vi "to and from repo test.vi"() -> ()   [LabVIEW 2013, in "configuration tests.lvlib"]
uses:
  configuration tests.lvlib
  Framework Configuration Classes/platypus configuration/targets cluster.ctl
  Framework Configuration Classes/target configuration/PL_Target Configuration.lvclass
  Framework Configuration Classes/platypus configuration/engines cluster.ctl
  <vilib>/NI/Module Execution Interface/Engine Configuration/engine configuration.lvclass
  <vilib>/NI/Tag Bus Module Framework/module configuration/TBM module configuration.lvclass
  Framework Configuration Classes/platypus configuration/systems cluster.ctl
  Framework Configuration Classes/system configuration/PL_System Configuration.lvclass
  Configuration Editor/Classes/SystemConfigRepo/SystemConfigRepo.lvclass
  Framework Configuration Classes/class cache/cache definition.ctl
  Framework Configuration Classes/class cache/cache search configuration.ctl
  Framework Configuration Classes/class cache/cached class information.ctl
  Framework Configuration Classes/class cache/target class metadata.ctl
  Framework Configuration Classes/class cache/class metadata.ctl
  <vilib>/NI/Tag Bus Module Framework/root configuration/Target Types.ctl
  <vilib>/NI/Tag Bus/tag/Data Type.ctl
  <vilib>/NI/Tag Bus/tag/tag descriptor.lvclass
  <vilib>/NI/Configuration Framework/serializable configuration/NISE_CEF_serializable configuration.lvclass/NISE_CEF_serializable configuration.ctl
  <vilib>/NI/Configuration Framework/serializable configuration/NISE_CEF_serializable configuration.lvclass
  Framework Configuration Classes/target configuration/PL_Target Configuration.lvclass/PL_Target Configuration.ctl
  Framework Configuration Classes/system configuration/PL_System Configuration.lvclass/PL_System Configuration.ctl
  test module/module/configuration/TEST CONFIGURATION.lvclass
  test module/module/configuration/state module configuration.ctl
  <vilib>/NI/Tag Bus Module Framework/channel/TBM channel.lvclass
  test module/module/configuration/TEST CONFIGURATION.lvclass/TEST CONFIGURATION.ctl
  Configuration Editor/Classes/SystemConfigRepo/SystemConfigRepo.lvclass/SystemConfigRepo.ctl
  <vilib>/NI/Tag Bus/tag/tag descriptor.lvclass/tag descriptor.ctl
  test module/module/configuration/Write state module configuration.vi
  test module/module/configuration/Read state module configuration.vi
  <vilib>/NI/Tag Bus/tag/read tag name.vi
  Framework Configuration Classes/target configuration/Write name.vi
  Framework Configuration Classes/system configuration/Write Configuration Name.vi
  Framework Configuration Classes/system configuration/Write save time.vi
  Configuration Editor/Classes/SystemConfigRepo/Write Systems.vi
  Configuration Editor/Classes/SystemConfigRepo/Read Systems.vi
  Framework Configuration Classes/system configuration/Read Configuration Name.vi
  Framework Configuration Classes/system configuration/Read save time.vi
  Framework Configuration Classes/target configuration/Read name.vi
  Framework Configuration Classes/platypus configuration/PLConfigurationSerializer.lvlib
  Framework Configuration Classes/class cache/PL_class cache.lvlib
  <vilib>/NI/Tag Bus Module Framework/root configuration/TBM configuration.lvclass
panel:
  out "moduleok":bool
  out "engok":bool
  out "engclasserr":errorcluster
  out "targok":bool
  out "sysok":bool
  # "THIS TEST FAILS WITHOUT A SAMPLE ENGINE IMPLEMENTATION"
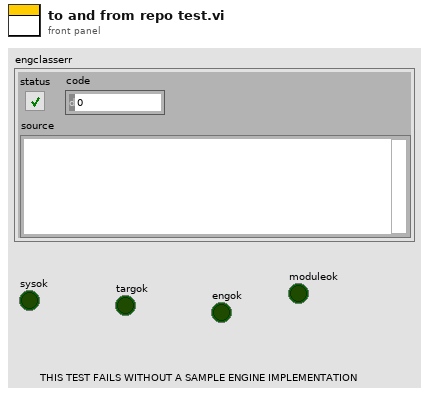
[diagram p1: front panel]
types:
  T1 = typedef "PLConfigurationSerializer.lvlib/engines cluster.ctl" = cluster{"engine configuration":refnum<class "engine configuration.lvclass">, "modules":refnum<class "TBM module configuration.lvclass">[]}
  T2 = typedef "PLConfigurationSerializer.lvlib/systems cluster.ctl" = cluster{"System Configuration":refnum<class "PL_System Configuration.lvclass">, "targets":T3[]}
  T3 = typedef "PLConfigurationSerializer.lvlib/targets cluster.ctl" = cluster{"Target Configuration":refnum<class "PL_Target Configuration.lvclass">, "engines":T1[]}
  T4 = typedef "PL_class cache.lvlib/cache definition.ctl" = cluster{"configuration":T5, "class cache data":T6}
  T5 = typedef "PL_class cache.lvlib/cache search configuration.ctl" = cluster{"Search Paths":path[], "Folders to Exclude":string[], "full class list":path[]}
  T6 = typedef "PL_class cache.lvlib/cached class information.ctl" = cluster{"targets":T7[], "engines":T8[], "modules":T8[], "ignored class list":path[]}
  T7 = typedef "PL_class cache.lvlib/target class metadata.ctl" = cluster{"file name":string, "fully qualified name":string, "menu display name":string, "configuration class name":string}
  T8 = typedef "PL_class cache.lvlib/class metadata.ctl" = cluster{"file name":string, "fully qualified name":string, "menu display name":string, "configuration class":string, "instances allowed":i32, "supported targets":T9[]}
  T9 = typedef "TBM configuration.lvclass/Target Types.ctl" = enum16{"Windows", "Mac", "Linux", "Linux RT ARM", "VxWorks", "Pharlap", "Other", "Linux RT x64"}
  T10 = typedef "tag bus.lvlib/tag descriptor.lvclass/Data Type.ctl" = enum16{"Double", "Single", "I64", "I32", "I16", "I8", "U64", "U32", "U16", "U8", "Boolean", "String", "Array of Double", "Array of Single", "Array of I64", "Array of I32", "Array of I16", "Array of I8", "Array of U64", "Array of U32", "Array of U16", "Array of U8", "Array of Boolean", "Array of String"}
  T11 = typedef "configuration tests.lvlib/TEST CONFIGURATION.lvclass/state module configuration.ctl" = cluster{"fixed input":refnum<class "TBM channel.lvclass">, "fixed output":refnum<class "TBM channel.lvclass">, "initial state":u8}
  T12 = typedef "NISE_CEF_Node.lvclass/NodeRef.ctl" = refnum<data-value>
  T13 = typedef "user tag bus module configuration.lvclass/state module configuration.ctl" = cluster{"fixed input":refnum<class "TBM channel.lvclass">, "fixed output":refnum<class "TBM channel.lvclass">, "initial state":u8}
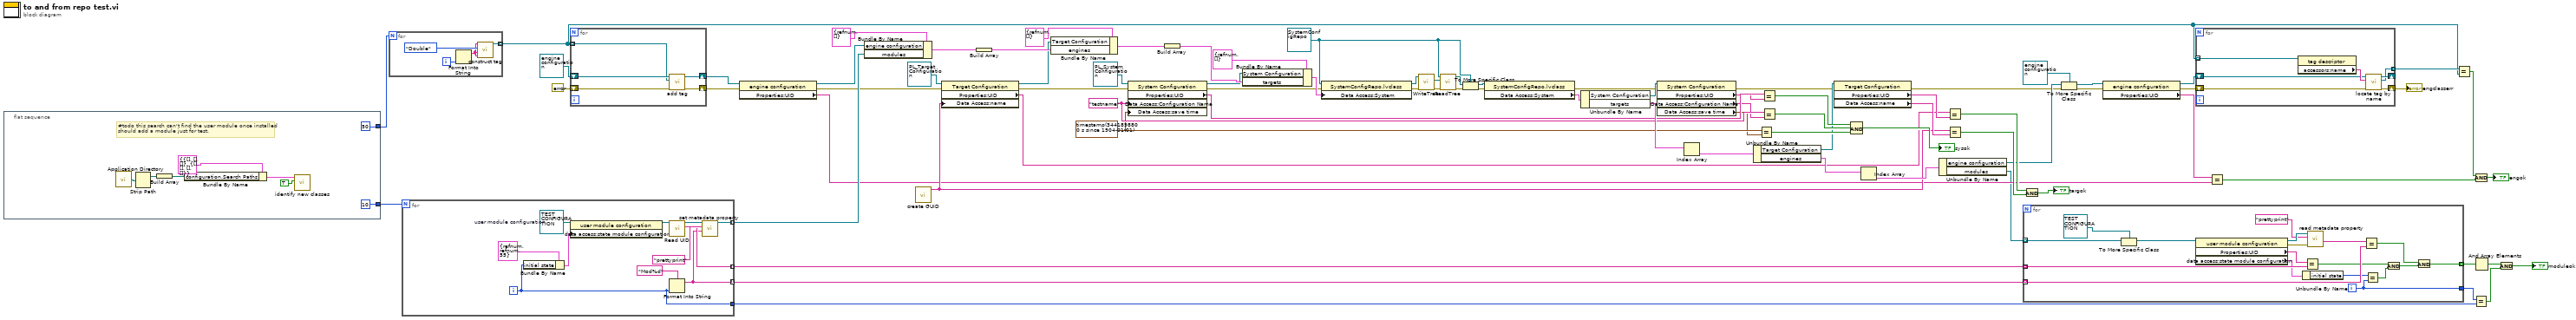
[diagram p0: block diagram]
diagram:
  w26 = refnum<class "SystemConfigRepo.lvclass"> refnum ("SystemConfigRepo in")
  w62 = timestamp(3441898800 s since 1904-01-01) ("save time")
  w63 = "testname" ("Configuration Name")
  n1 = flat-sequence {
    tunnel: [10] -> w22
    tunnel: [50] -> w1
    frame #0 {
      # "#todo this search can't find the user module once installed\nshould add a module just for test."
      n2 = call <vilib>:"Application Directory.vi"() -> ("Application Directory"=w83:path)
      n3 = Strip Path(path=w83) -> (stripped path=w84:path)  [unwired: 1 out]
      n4 = Build Array(w84) -> (w85:path[])
      n5 = Bundle By Name(cluster=T4 {"configuration"={"Search Paths"=[], "Folders to Exclude"=[], "full class list"=[]}, "class cache data"={"targets"=[], "engines"=[], "modules"=[], "ignored class list"=[]}} ("cache"), "configuration.Search Paths"=w85) -> (w89:T4)
      n6 = call "identify new classes.vi"("force scan"=TRUE, "cache in"=w89) -> ()  [unwired: 8 in, 2 out]
    }
  }
  n7 = for {
    N: w1 -> [_]
    tunnel: [w91] -> w6 mode=indexing
    i -> [w94]
    n8 = Format Into String(w94) -> (resulting string=w92:string)  [unwired: 3 in, 1 out]
    n9 = call <vilib>:"construct tag.vi"("raw default"=w92, "metadata"=w92, "data type"=Data_Type."Double", "name"=w92) -> ("system tag out"=w91:refnum<class "tag descriptor.lvclass">)  [unwired: 6 in, 1 out]
  }
  n10 = for {
    N: w22 -> [_]
    tunnel: [w103] -> w75 mode=indexing
    tunnel: [w101] -> w36 mode=indexing
    tunnel: [w100] -> w37 mode=indexing
    tunnel: [w95] -> w2
    i -> [w95]
    w99 = refnum<class "TEST CONFIGURATION.lvclass"> refnum  # user module configuration
    n11 = Bundle By Name(cluster=T11 {"fixed input"=refnum, "fixed output"=refnum, "initial state"=55} ("state module configuration"), "initial state"=w95) -> (w96:T11)
    n12 = property class="user module configuration"(reference=w99, "data access:state module configuration"=w96) -> (reference out=w98:refnum<class "TEST CONFIGURATION.lvclass">)  [unwired: 1 in, 1 out]
    n13 = call <vilib>:"Read UID.vi"("configuration in"=w98) -> ("instance id"=w101:string, "configuration out"=w104:refnum<class "TEST CONFIGURATION.lvclass">)  [unwired: 8 in, 1 out]
    n14 = Format Into String(format string="Mod%d", w95) -> (resulting string=w100:string)  [unwired: 2 in, 1 out]
    n15 = call <vilib>:"set metadata property.vi"("value"=w100, "key"="prettyprint", "configuration in"=w104) -> ("configuration out"=w103:refnum<class "TEST CONFIGURATION.lvclass">)  [unwired: 7 in, 1 out]
  }
  n16 = for {
    shift-right: [w110] -> w10
    shift-left: refnum<class "engine configuration.lvclass"> refnum ("Engine Configuration") -> [w109]
    shift-right: [w108] -> w8
    shift-left: errorcluster {"status"=FALSE, "code"=0, "source"=""} ("error out") -> [w107]
    tunnel: w6 -> [w106] mode=indexing
    n17 = call <vilib>:"add tag.vi"("error in"=w107, "tag descriptor"=w106, "engine configuration in"=w109) -> ("error out"=w108:errorcluster, "engine configuration out"=w110:refnum<class "engine configuration.lvclass">)  [unwired: 7 in]
  }
  n18 = property class="engine configuration"(reference=w10, error in=w8) -> (reference out=w74:refnum<class "engine configuration.lvclass">, error out=w17:errorcluster, "Properties:UID"=w39:string)
  n19 = Bundle By Name(cluster=T1 {"engine configuration"=refnum, "modules"=[]} ("engines cluster"), "engine configuration"=w74, "modules"=w75) -> (w81:T1)
  n20 = call <vilib>:"create GUID.vi"() -> ("uuid"=w48:string)  [unwired: 11 in]
  n21 = property class="Target Configuration"(reference=refnum<class "PL_Target Configuration.lvclass"> refnum ("Target Configuration"), error in=w17, "Data Access:name"=w48) -> (reference out=w72:refnum<class "PL_Target Configuration.lvclass">, error out=w16:errorcluster, "Properties:UID"=w47:string)
  n22 = Build Array(w81) -> (w79:T1[])
  n23 = Bundle By Name(cluster=T3 {"Target Configuration"=refnum, "engines"=[]} ("targets cluster"), "Target Configuration"=w72, "engines"=w79) -> (w78:T3)
  n24 = property class="System Configuration"(reference=refnum<class "PL_System Configuration.lvclass"> refnum ("System Configuration"), error in=w16, "Data Access:Configuration Name"=w63, "Data Access:save time"=w62) -> (reference out=w70:refnum<class "PL_System Configuration.lvclass">, error out=w18:errorcluster, "Properties:UID"=w64:string)
  n25 = Build Array(w78) -> (w76:T3[])
  n26 = Bundle By Name(cluster=T2 {"System Configuration"=refnum, "targets"=[]} ("system"), "System Configuration"=w70, "targets"=w76) -> (w31:T2)
  n27 = property class="SystemConfigRepo.lvclass"(reference=w26, error in=w18, "Data Access:System"=w31) -> (reference out=w33:refnum<class "SystemConfigRepo.lvclass">, error out=w32:errorcluster)
  n28 = call-dynamic "WriteTree.vi"("error in"=w32, "SystemConfigRepo in"=w33) -> ("error out"=w30:errorcluster, "root"=w29:T12)  [unwired: 7 in, 1 out]
  n29 = call-dynamic "ReadTree.vi"("error in"=w30, "root"=w29, "SystemConfigRepo in"=w26) -> ("error out"=w23:errorcluster, "repository out"=w28:refnum<class "NISE_CEF_Repository.lvclass">)  [unwired: 7 in]
  n30 = To More Specific Class(target class=w26, reference=w28, error in=w23) -> (specific class reference=w27:refnum<class "SystemConfigRepo.lvclass">, error out=w24:errorcluster)
  n31 = property class="SystemConfigRepo.lvclass"(reference=w27, error in=w24) -> (error out=w19:errorcluster, "Data Access:System"=w25:T2)  [unwired: 1 out]
  n32 = Unbundle By Name(w25) -> ("System Configuration"=w65:refnum<class "PL_System Configuration.lvclass">, "targets"=w69:T3[])
  n33 = property class="System Configuration"(reference=w65, error in=w19) -> (error out=w20:errorcluster, "Properties:UID"=w59:string, "Data Access:Configuration Name"=w60:string, "Data Access:save time"=w61:timestamp)  [unwired: 1 out]
  n34 = Index Array(array=w69) -> (element=w67:T3)  [unwired: 1 in]
  n35 = Unbundle By Name(w67) -> ("Target Configuration"=w54:refnum<class "PL_Target Configuration.lvclass">, "engines"=w68:T1[])
  n36 = Equal?(x=w62, y=w61) -> (x = y?=w56:bool)
  n37 = Equal?(x=w64, y=w59) -> (x = y?=w58:bool)
  n38 = Equal?(x=w63, y=w60) -> (x = y?=w57:bool)
  n39 = property class="Target Configuration"(reference=w54, error in=w20) -> (error out=w21:errorcluster, "Properties:UID"=w49:string, "Data Access:name"=w50:string)  [unwired: 1 out]
  n40 = Compound Arithmetic op=AND(w58, w57, w56) -> (→"sysok":bool)
  n41 = Index Array(array=w68) -> (element=w66:T1)  [unwired: 1 in]
  n42 = Unbundle By Name(w66) -> ("engine configuration"=w46:refnum<class "engine configuration.lvclass">, "modules"=w38:refnum<class "TBM module configuration.lvclass">[])
  n43 = Equal?(x=w47, y=w49) -> (x = y?=w51:bool)
  n44 = Equal?(x=w48, y=w50) -> (x = y?=w52:bool)
  n45 = for {
    tunnel: w38 -> [w128] mode=indexing
    tunnel: w37 -> [w123] mode=indexing
    tunnel: w36 -> [w121] mode=indexing
    tunnel: [w119] -> w35 mode=indexing
    tunnel: [w111] -> w4
    i -> [w111]
    n46 = To More Specific Class(target class=refnum<class "TEST CONFIGURATION.lvclass"> refnum ("user module configuration"), reference=w128) -> (specific class reference=w118:refnum<class "TEST CONFIGURATION.lvclass">)  [unwired: 1 in, 1 out]
    n47 = property class="user module configuration"(reference=w118) -> (reference out=w127:refnum<class "TEST CONFIGURATION.lvclass">, error out=w125:errorcluster, "Properties:UID"=w122:string, "data access:state module configuration"=w116:T13)  [unwired: 1 in]
    n48 = Unbundle By Name(w116) -> ("initial state"=w113:u8)
    n49 = Equal?(x=w122, y=w121) -> (x = y?=w115:bool)
    n50 = call <vilib>:"read metadata property.vi"("error in"=w125, "key"="prettyprint", "configuration in"=w127) -> ("value"=w124:string)  [unwired: 5 in, 3 out]
    n51 = Equal?(x=w124, y=w123) -> (x = y?=w120:bool)
    n52 = Equal?(x=w113, y=w111) -> (x = y?=w112:bool)
    n53 = And(x=w115, y=w112) -> (x .and. y?=w114:bool)
    n54 = And(x=w120, y=w114) -> (x .and. y?=w119:bool)
  }
  n55 = Compound Arithmetic op=AND(w51, w52) -> (→"targok":bool)
  n56 = To More Specific Class(target class=refnum<class "engine configuration.lvclass"> refnum ("Engine Configuration"), reference=w46, error in=w21) -> (specific class reference=w45:refnum<class "engine configuration.lvclass">, error out=w44:errorcluster)
  n57 = property class="engine configuration"(reference=w45, error in=w44) -> (reference out=w12:refnum<class "engine configuration.lvclass">, error out=w14:errorcluster, "Properties:UID"=w40:string)
  n58 = for {
    shift-right: [w134] -> w13
    shift-left: w14 -> [w135]
    tunnel: w6 -> [w133] mode=indexing
    shift-right: [w131] -> _
    shift-left: w12 -> [w130]
    tunnel: [w129] -> w11 mode=indexing
    n59 = property class="tag descriptor"(reference=w133) -> ("accessors:name"=w132:string)  [unwired: 1 in, 2 out]
    n60 = call <vilib>:"locate tag by name.vi"("error in"=w135, "tag name"=w132, "engine configuration in"=w130) -> ("error out"=w134:errorcluster, "tag descriptor"=w129:refnum<class "tag descriptor.lvclass">, "engine configuration out"=w131:refnum<class "engine configuration.lvclass">)  [unwired: 6 in]
  }
  "engclasserr" <- w13
  n61 = Equal?(x=w40, y=w39) -> (x = y?=w42:bool)
  n62 = Equal?(x=w11, y=w6) -> (x = y?=w43:bool)
  n63 = And Array Elements(Boolean array=w35) -> (logical AND=w34:bool)
  n64 = Equal?(x=w4, y=w2) -> (x = y?=w3:bool)
  n65 = Compound Arithmetic op=AND(w43, w42) -> (→"engok":bool)
  n66 = And(x=w34, y=w3) -> (x .and. y?=→"moduleok":bool)
